vi "Main Loop.vi"(8 "error in (no error)":errorcluster, 10 "Chart Notifier":refnum<notifier>, 11 "Message Queues":T1) -> (0 "error out":errorcluster)   [LabVIEW 2018, in "Scale Module.lvlib" / "Scale Module Engine.lvlib"]
uses:
  Scale Module Engine.lvlib
  Scale Message Queues.ctl
  support/Message Queue/Message Cluster.ctl
  State Cluster.ctl
  State Enum.ctl
  Feed Module/Controls/Scale Module Settings Cluster.ctl
  Mettler Toledo/Controls/Settings Cluster.ctl
  Feed Module/Controls/Scale Module Display.ctl
  <vilib>/Platform/TimedLoop/XDataNode/timing_clust.ctl
  <vilib>/Platform/TimedLoop/XDataNode/nitl_modes.ctl
  <vilib>/Platform/TimedLoop/XDataNode/wakeup.ctl
  Tag VIs/Tag FGV Operation Enum.ctl
  support/Message Queue/Enqueue Message (Single).vi
  <vilib>/Platform/TimedLoop/XDataNode/XDataNode.xnode
  support/Message Queue/Message Queue.lvlib
  <vilib>/Platform/TimedLoop/XDataNode/XDNodeRunTimeDep.lvlib
  Scale Module.lvlib
  Mettler Toledo/Mettler Toledo.lvlib
  Shared Variables/Dynamic Shared Variables.lvlib
  support/Support Library.lvlib
panel:
  out "Period (s)":dbl format="%_4g"
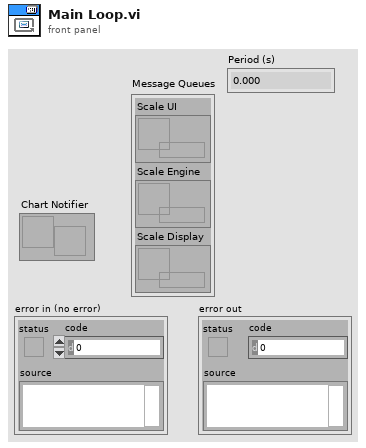
[diagram p1: front panel]
types:
  T1 = typedef "Scale Module.lvlib/Scale Message Queues.ctl" = cluster{"Scale UI":refnum<queue>, "Scale Engine":refnum<queue>, "Scale Display":refnum<queue>}
  T2 = typedef "Scale Module.lvlib/Scale Module Engine.lvlib/State Cluster.ctl" = cluster{"State":T3, "Start Time":timestamp, "Configuration":T4, "Current Time":timestamp, "First Iteration":bool, "Data":cluster{"Scale Read(g)":dbl}, "Process Name":string, "Log Started":bool}
  T3 = typedef "Scale Module.lvlib/Scale Module Engine.lvlib/State Enum.ctl" = enum16{"Measuring", "Idle"}
  T4 = typedef "Scale Module.lvlib/Scale Module Settings Cluster.ctl" = cluster{"Cycle Period":dbl, "Mettler":T5, "Scale Type":string}
  T5 = typedef "Mettler Toledo.lvlib/Settings Cluster.ctl" = cluster{"VISA resource name":refnum<visa-resource-name>, "Simulated?":bool}
  T6 = typedef "XDNodeRunTimeDep.lvlib/timing_clust.ctl" = cluster{"Expected End [f-1]":u64, "Actual End [f-1]":u64, "Finished Late? [f-1]":bool, "Expected End [i-1]":u64, "Actual End [i-1]":u64, "Finished Late? [i-1]":bool, "Expected Start [i]":u64, "Actual Start [i]":u64, "Expected Start [f]":u64, "Actual Start [f]":u64, "Source Name":string, "Structure Name":string, "Period":i64, "Deadline":i64, "Offset":i64, "Start":i64, "Priority":i32, "Timeout":i32, "Mode":T7, "Wakeup Reason":T8, "Error":errorcluster, "Source Type":string, "Secondary Source Type":string, "Global End Time":u64, "Global Start Time":u64, "Frame Duration":u64, "Iteration Duration":u64, "Assigned CPU":i32, "I/O Scan Engine Mode":u32}
  T7 = typedef "XDNodeRunTimeDep.lvlib/nitl_modes.ctl" = enum32{"No Change", "Process missed periods, maintain original phase", "Discard missed periods, maintain original phase", "Process missed periods, ignore original phase", "Discard missed periods, ignore original phase"}
  T8 = typedef "XDNodeRunTimeDep.lvlib/wakeup.ctl" = enum32{"Normal", "Aborted", "Asynchronous wakeup", "Timing source error", "Timed loop error", "Timeout"}
  T9 = cluster{"enable? (F)":bool, "name":string, "alarm on":bool, "priority":u32, "ack type":enum16{"Auto", "User", "None", "Each Occurrence"}, "area":string, "description":string, "log? (T)":bool}
  T10 = typedef "Tag FGV Operation Enum.ctl" = enum16{"Init", "Set Notification Queue", "Create Tag", "Commit", "Write Tag (Numeric)", "Write Tag (Boolean)", "Read All Tags", "Read One Tag", "Delete Tag Category", "Set Alarm Parameters (Numeric)", "Set Alarm Parameters (Boolean)", "Enable All Alarms", "Disable All Alarms", "Delete All Tags", "Read Alarms", "Ack Alarm", "Read Alarm Parameters (Numeric)", "Read Alarm Parameters (Boolean)"}
  T11 = enum32{"u32BitField", "bool", "double", "string", "int8", "uint8", "int16", "uint16", "int32", "uint32", "int64", "uint64", "single", "double waveform", "int16 waveform", "array of boolean", "array of int8", "array of uint8", "array of int16", "array of uint16", "array of int32", "array of uint32", "array of int64", "array of uint64", "array of single", "array of double", "array of double waveform", "array of int16 waveform", "array of string", "variant", "timestamp", "fixed point", "custom"}
  T12 = typedef "Scale Module.lvlib/Scale Module Display.ctl" = cluster{"Scale Value":dbl, "Cycle Period":dbl}
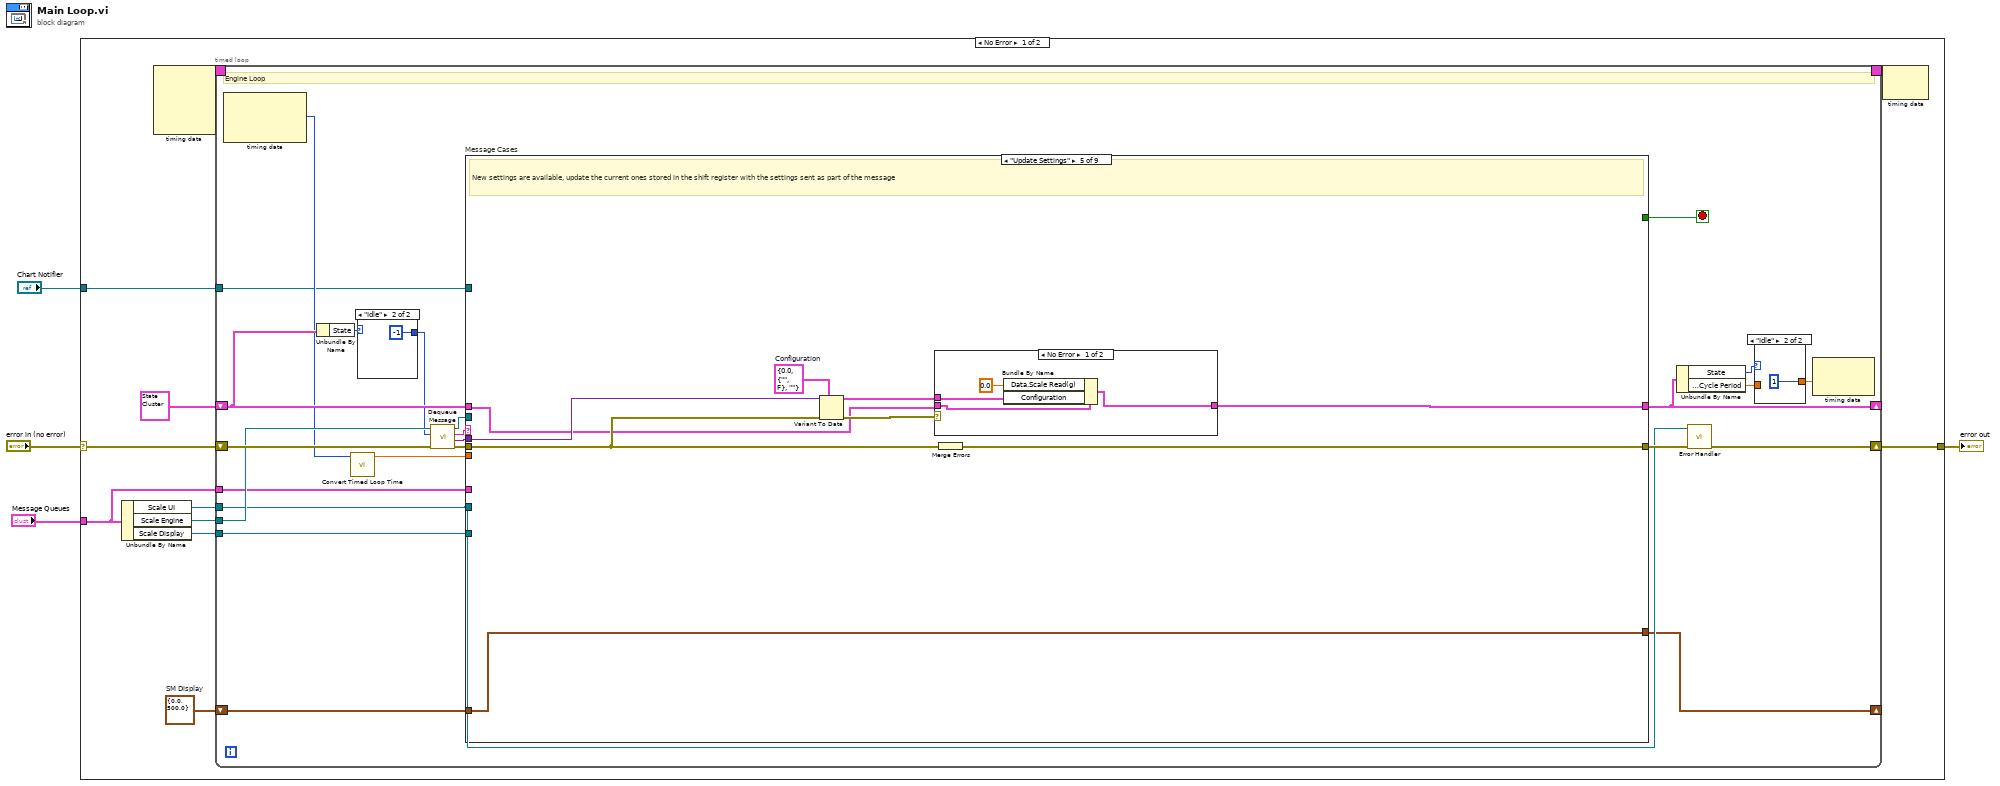
[diagram p0: block diagram]
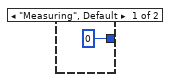
[diagram p3: hidden frame]
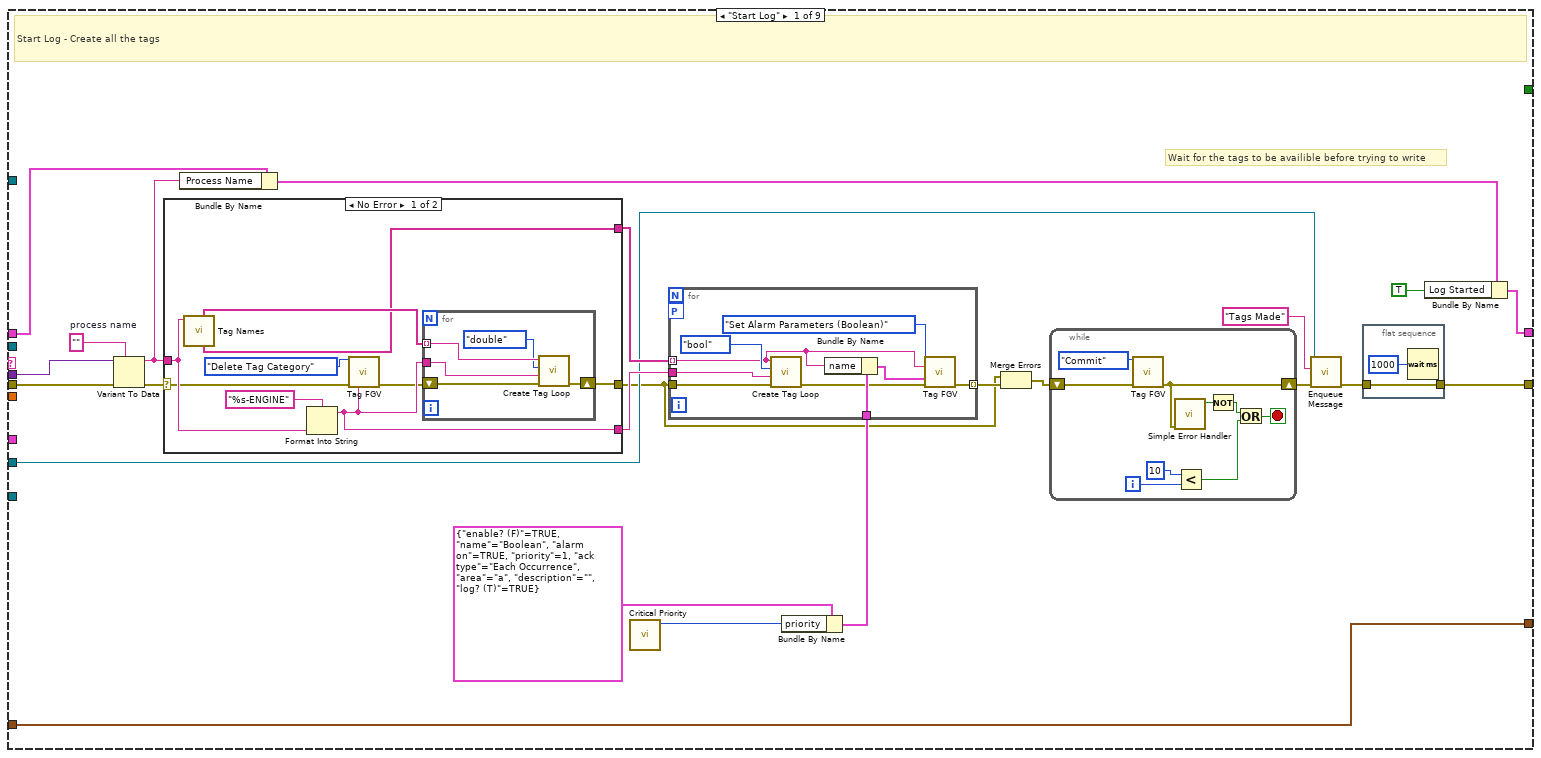
[diagram p4: hidden frame]
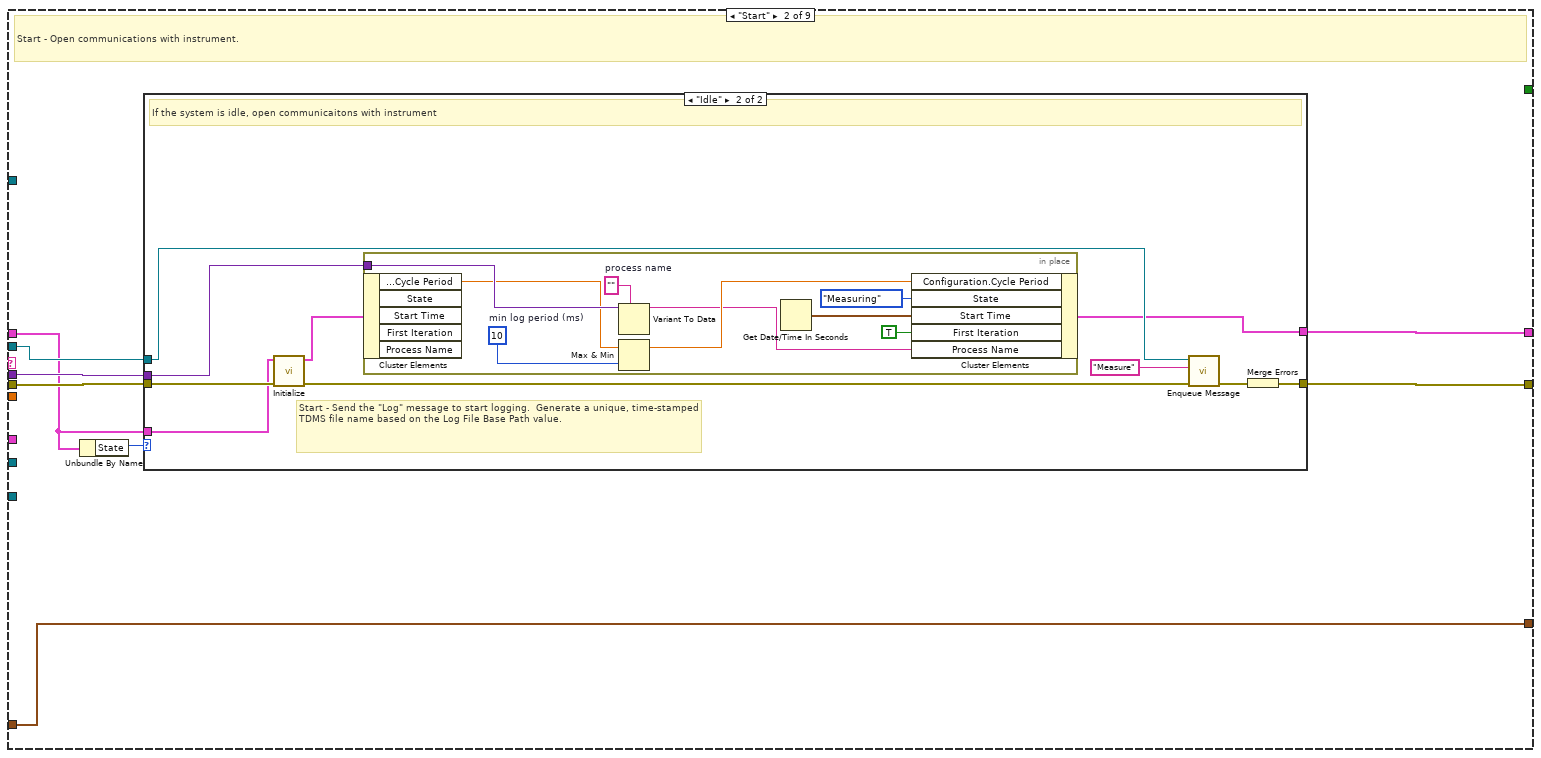
[diagram p6: hidden frame]
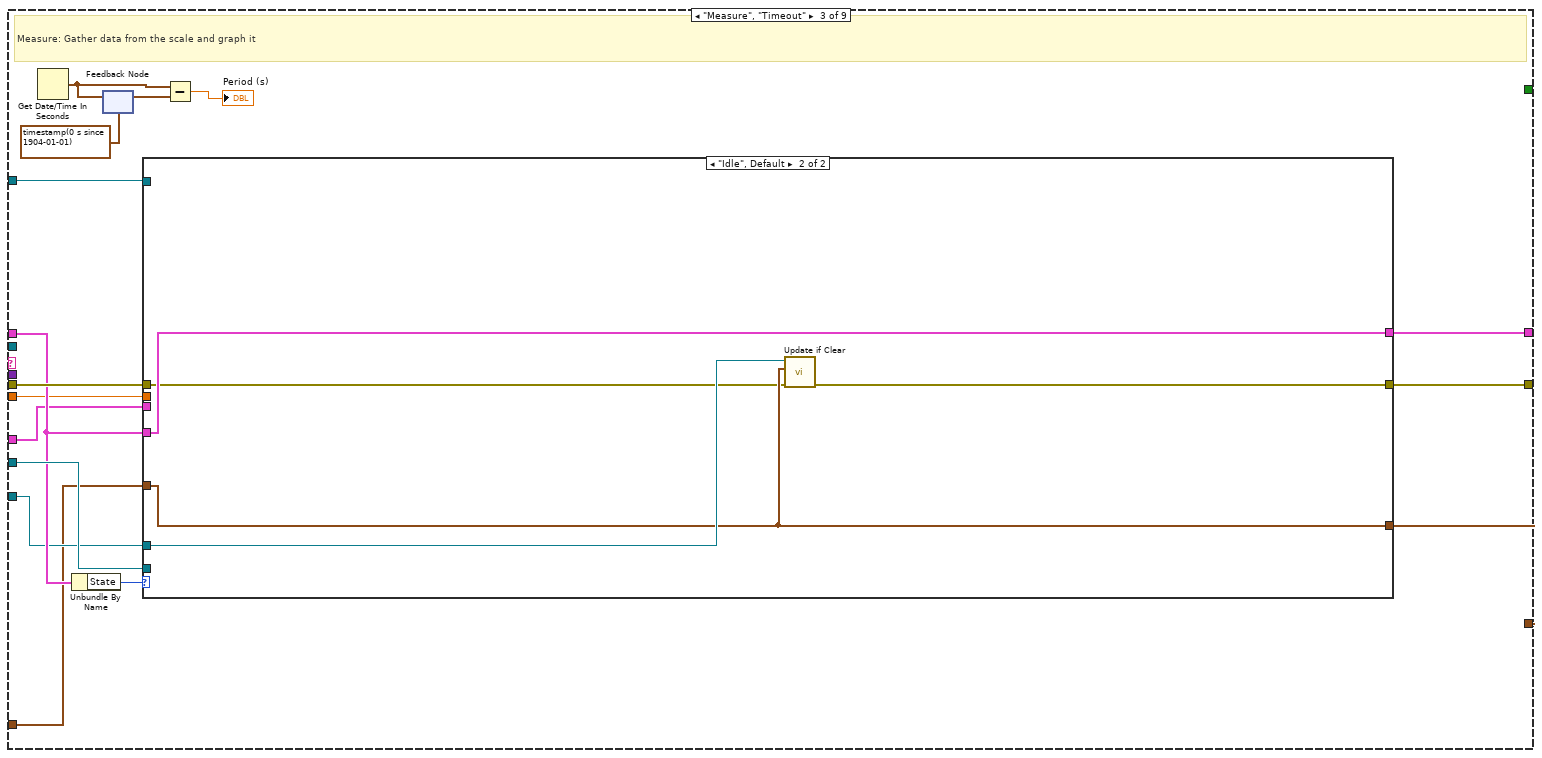
[diagram p8: hidden frame]
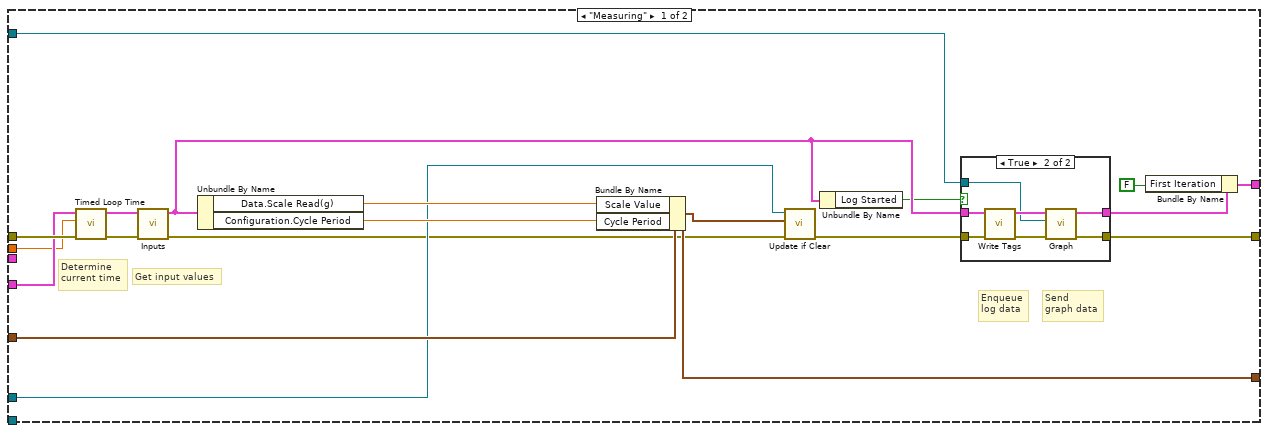
[diagram p9: hidden frame]
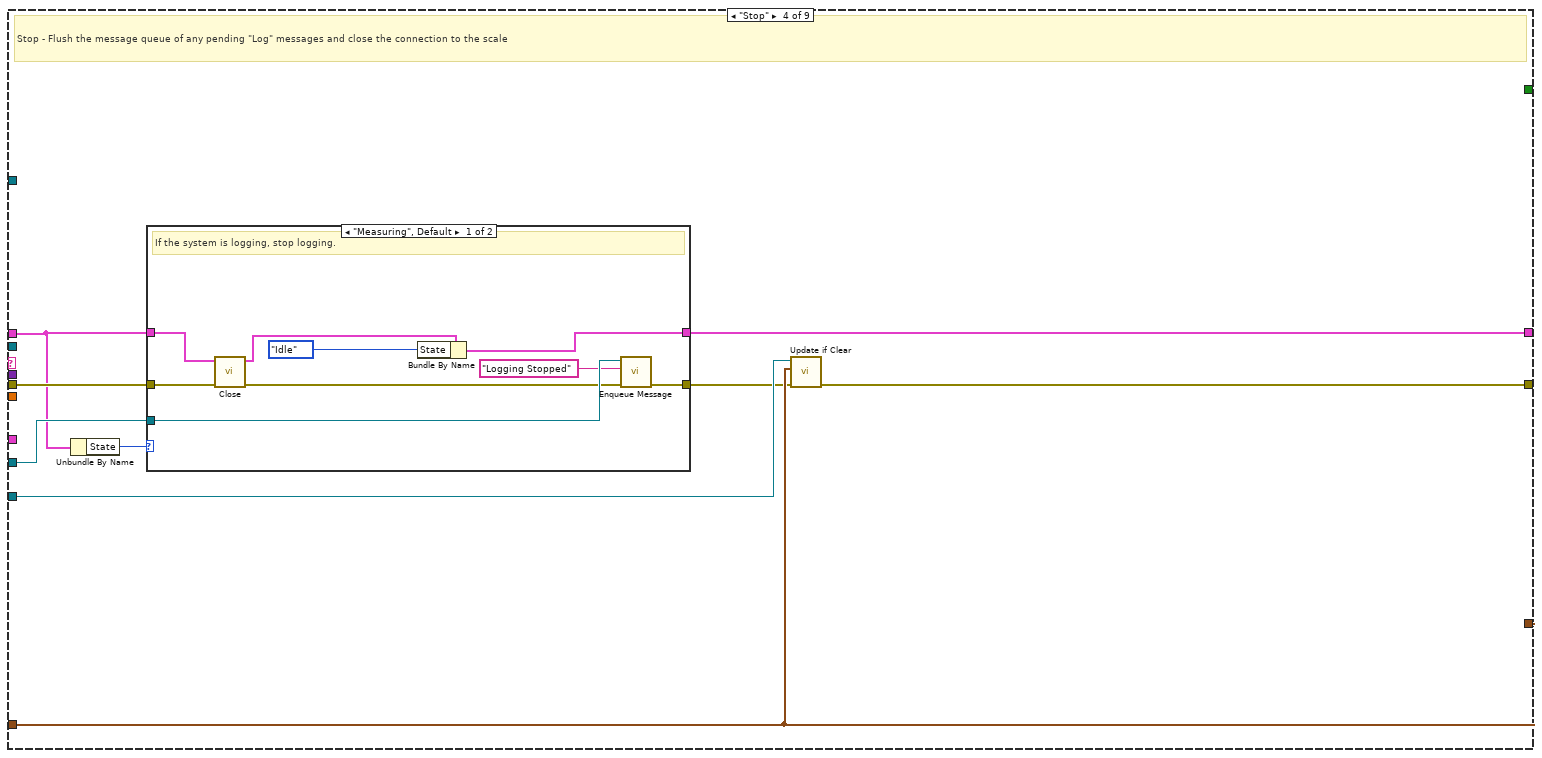
[diagram p11: hidden frame]
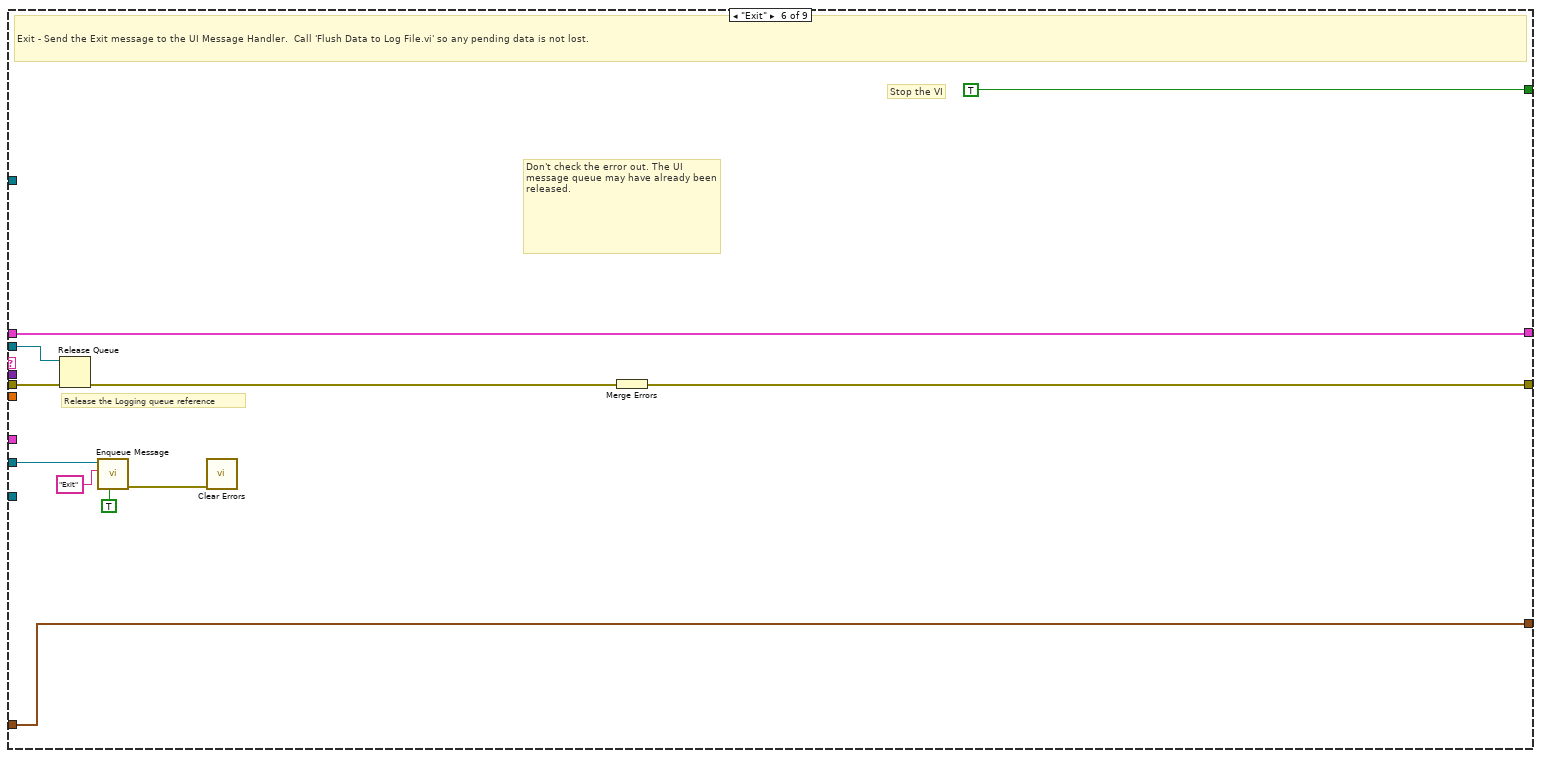
[diagram p14: hidden frame]
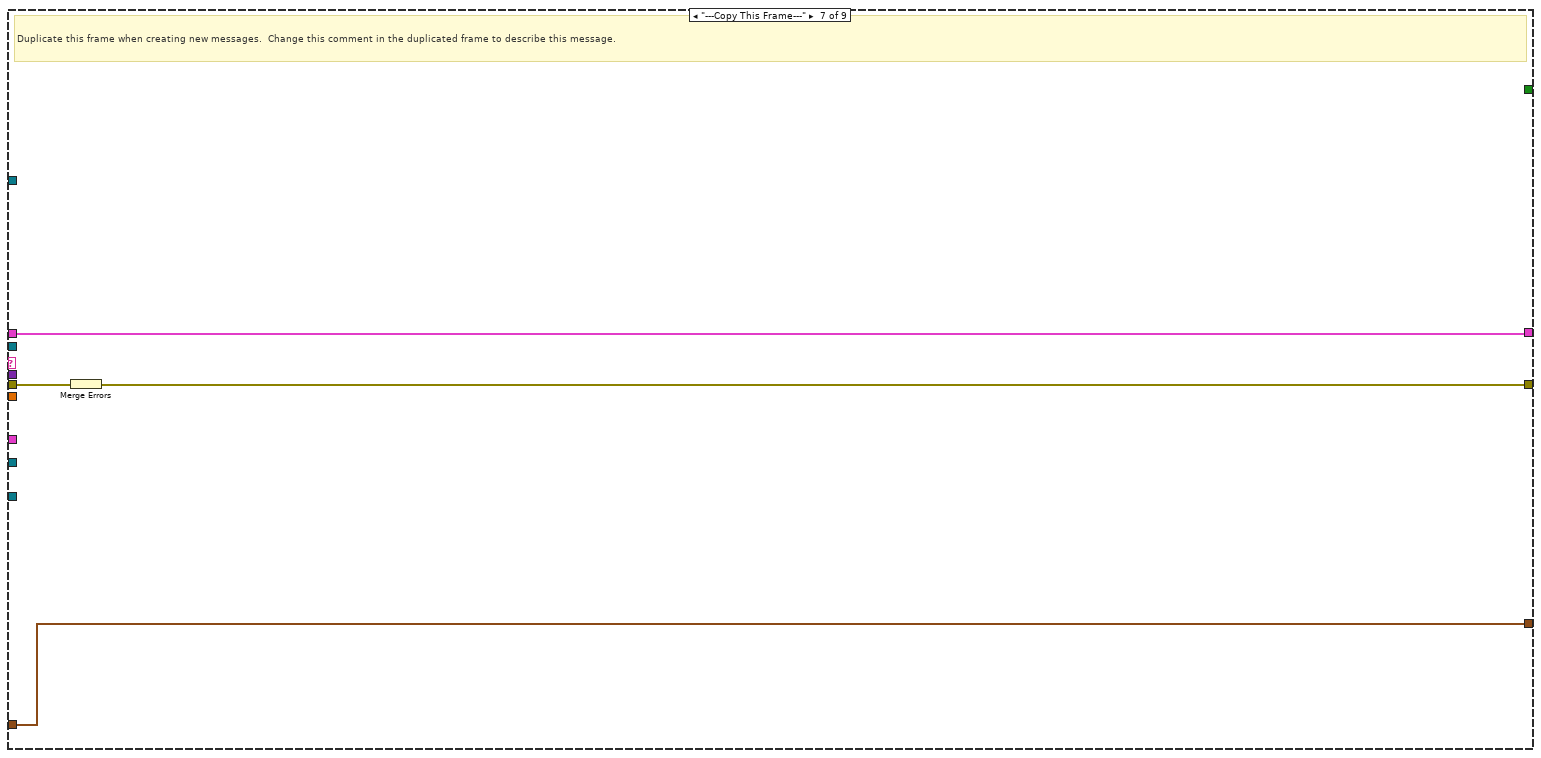
[diagram p15: hidden frame]
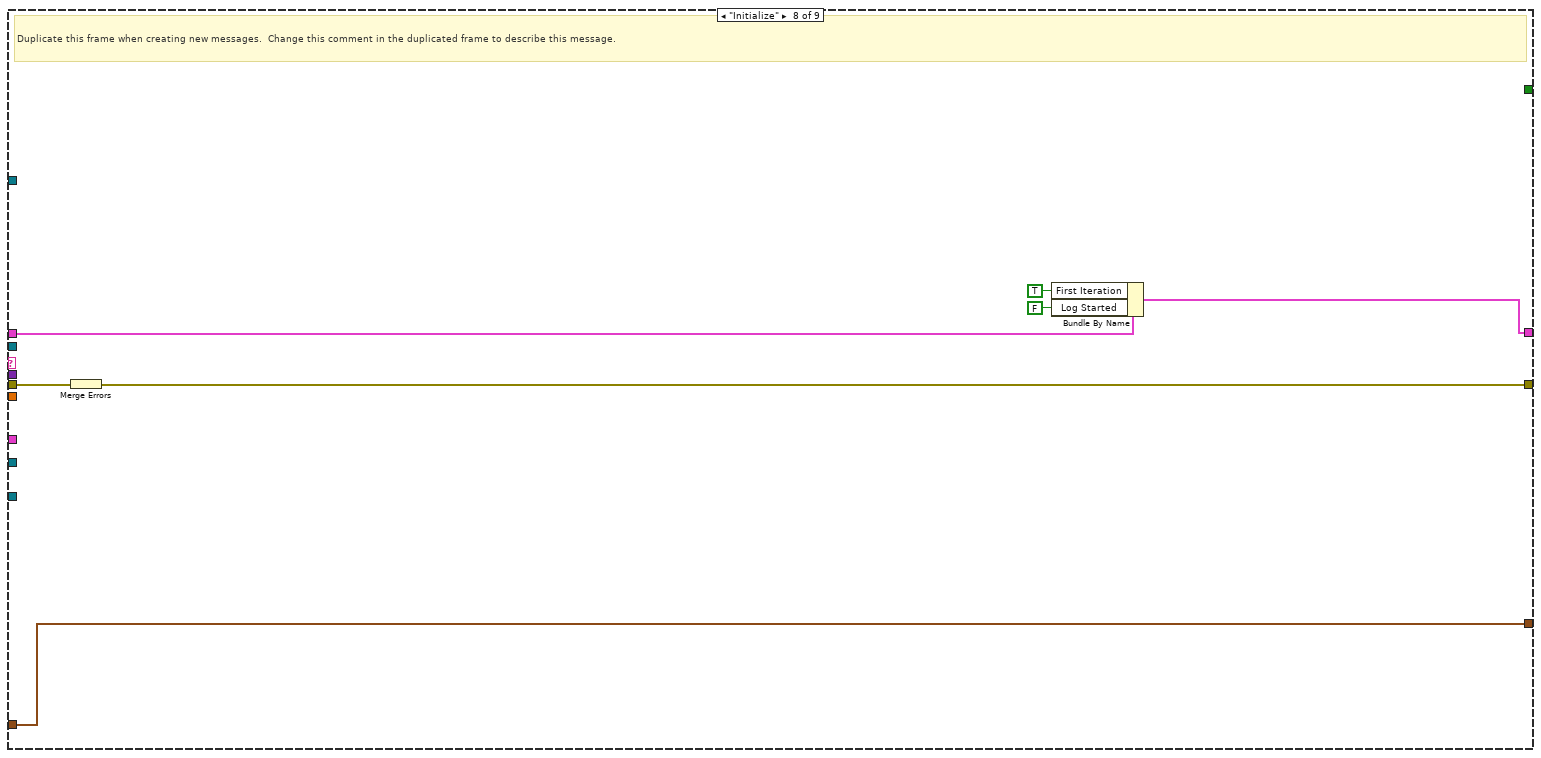
[diagram p16: hidden frame]
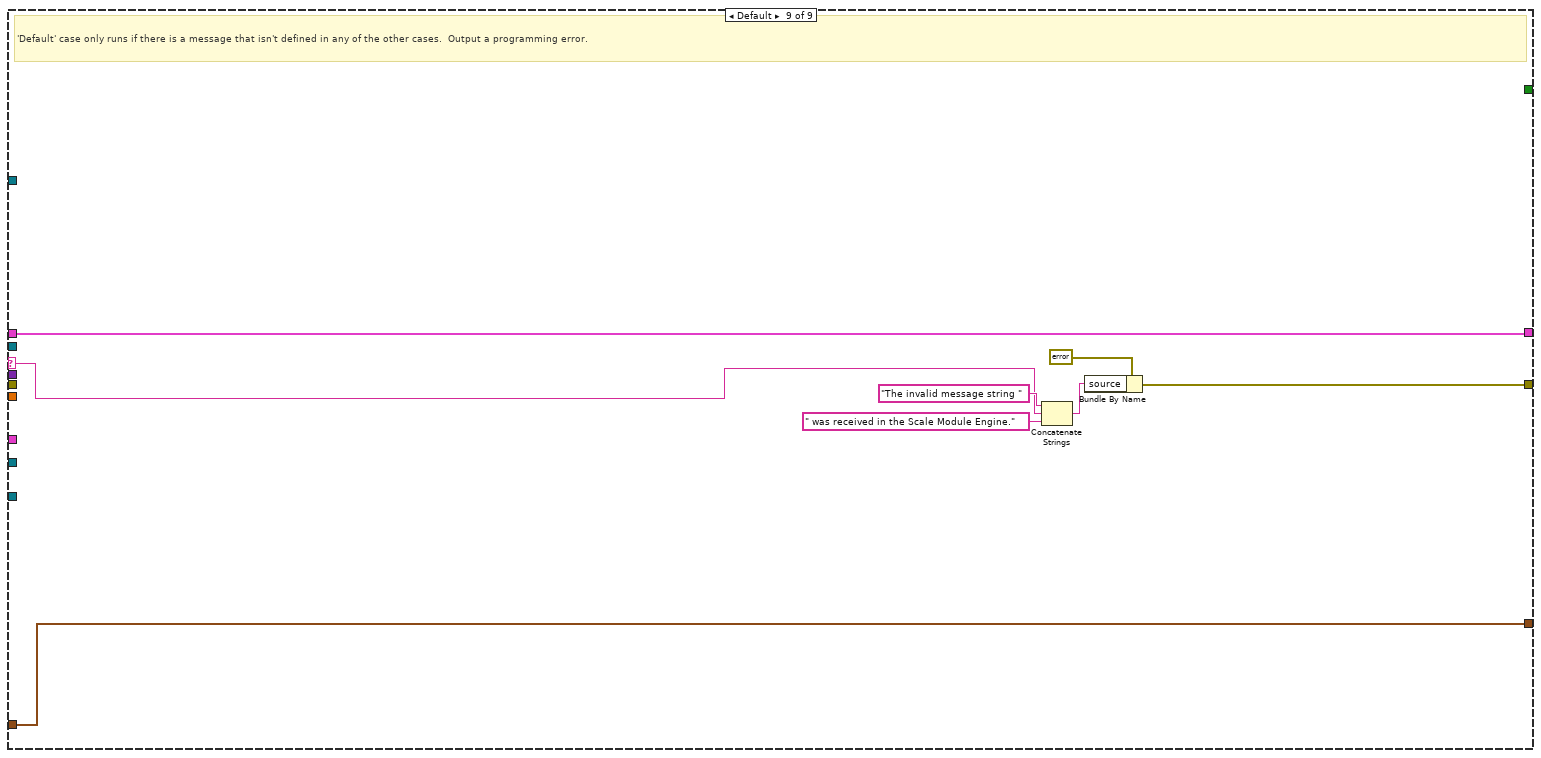
[diagram p17: hidden frame]
diagram:
  n1 = case shown="No Error" "error in (no error)" {
    selector: "error in (no error)" -> [w14 w251]
    tunnel: "Message Queues" -> [w9 _]
    tunnel: [w15 w251] -> w3
    tunnel: "Chart Notifier" -> [w7 _]
    frame No Error {
      w5 = T12 {"Scale Value"=0.0, "Cycle Period"=500.0}  # SM Display
      n2 = Unbundle By Name(w9) -> ("Scale UI"=w13:refnum<queue>, "Scale Engine"=w8:refnum<queue>, "Scale Display"=w6:refnum<queue>)
      n3 = node-c288() -> (w11:T6)  [unwired: 4 in]
      n4 = timed-loop {
        tunnel: w8 -> [w33]
        shift-right: [w17] -> _
        shift-left: T2 {"State"=enum."Idle", "Start Time"=timestamp(0 s since 1904-01-01), "Configuration"={"Cycle Period"=0.0, "Mettler"={"VISA resource name"="", "Simulated?"=FALSE}, "Scale Type"=""}, "Current Time"=timestamp(0 s since 1904-01-01), "First Iteration"=FALSE, "Data"={"Scale Read(g)"=0.0}, "Process Name"="", "Log Started"=FALSE} -> [w29]
        shift-right: [w31] -> w15
        shift-left: w14 -> [w38]
        tunnel: w13 -> [w30]
        timing: w11 -> [_]
        timing-out: [_] -> w10
        tunnel: w9 -> [w21]
        tunnel: w7 -> [w20]
        tunnel: w6 -> [w19]
        shift-right: [w18] -> _
        shift-left: w5 -> [w16]
        stop <- w39 stop-if-true
        # "Engine Loop"
        n5 = node-c288() -> (w23:i64)  [unwired: 1 in, 2 out]
        n6 = Unbundle By Name(w29) -> ("State"=w28:T3)
        n7 = call "Convert Timed Loop Time.vi"("Actual Start [i]"=w23) -> ("ET since start (s)"=w22:dbl)  [unwired: 10 in]
        n8 = case shown="\"Idle\"" w28 {
          tunnel: [0 ("timeout in ms (-1)") -1 ("timeout in ms (-1)")] -> w27
          frame "Measuring", Default {
          }
          frame "Idle" {
          }
        }
        n9 = call "Dequeue Message.vi"("error in (no error)"=w38, "timeout in ms (-1)"=w27, "Message Queue"=w33) -> ("error out"=w37:errorcluster, "Message Data"=w35:variant, "Message"=w36:string, "dup Message Queue"=w34:refnum<queue>)  [unwired: 5 in]
        n10 = case "Message Cases" shown="\"Update Settings\"" w36 {
          selector: w36 -> [_ _ _ _ _ _ _ _ w242]
          tunnel: w34 -> [_ w113 _ _ _ w223 _ _ _]
          tunnel: w37 -> [w66 w112 w148 w193 w211 w226 w233 w240 _]
          tunnel: [w50 w114 w149 w185 w213 w228 w232 w239 w241] -> w32
          tunnel: w29 -> [w65 w109 w147 w190 w209 w219 w230 w237 w247]
          tunnel: [_ _ _ _ _ TRUE _ _ _] -> w39
          tunnel: w35 -> [w67 w110 _ _ w212 _ _ _ _]
          tunnel: w30 -> [w54 _ w150 w192 _ w227 _ _ _]
          tunnel: w22 -> [_ _ w146 _ _ _ _ _ _]
          tunnel: w21 -> [_ _ w145 _ _ _ _ _ _]
          tunnel: w20 -> [_ _ w141 _ _ _ _ _ _]
          tunnel: w19 -> [_ _ w140 w188 _ _ _ _ _]
          tunnel: w16 -> [w71 w108 w139 w187 w206 w220 w231 w238 w248]
          tunnel: [w71 w108 w138 w187 w206 w220 w231 w238 w248] -> w18
          tunnel: [w57 w107 w137 w189 w205 w219 w230 w234 w247] -> w17
          frame "Start Log" {
            w70 = ""  # process name
            # "Wait for the tags to be availible before trying to write"
            # "Start Log - Create all the tags"
            n11 = Variant To Data(error in=w66, type=w70, Variant=w67) -> (data=w68:string, error out=w69:errorcluster)
            n12 = case shown="No Error" w69 {
              selector: w69 -> [w94 w106]
              tunnel: [w100 w106] -> w49
              tunnel: w68 -> [w98 _]
              tunnel: [w93 _] -> w61
              tunnel: [w96 _] -> w60
              frame No Error {
                n13 = call "Tag Names.vi"("Process Name"=w98) -> ("All Boolean Tags"=w96:string[], "All  Numeric Tags"=w97:string[])  [unwired: 8 in, 1 out]
                n14 = Format Into String(format string="%s-ENGINE", w98) -> (resulting string=w93:string)  [unwired: 2 in, 1 out]
                n15 = call "Tag FGV.vi"("Operation"=Tag_FGV_Operation_Enum."Delete Tag Category", "error in (no error)"=w94, "Tag Category"=w93) -> ("error out"=w92:errorcluster)  [unwired: 5 in, 7 out]
                n16 = for {
                  shift-right: [w105] -> w100
                  shift-left: w92 -> [w104]
                  tunnel: w93 -> [w101]
                  tunnel: w97 -> [w103] mode=indexing
                  n17 = call "Create Tag Loop.vi"("error in (no error)"=w104, "Tag Category"=w101, "data type"=T11."double", "Tag Name"=w103) -> ("error out"=w105:errorcluster)  [unwired: 7 in]
                }
              }
              frame Error {
              }
            }
            n18 = Bundle By Name(cluster=w65, "Process Name"=w68) -> (w58:T2)
            n19 = call "Critical Priority.vi"() -> ("critical priority"=w63:i32)  [unwired: 11 in]
            n20 = Bundle By Name(cluster=T9 {"enable? (F)"=TRUE, "name"="Boolean", "alarm on"=TRUE, "priority"=1, "ack type"=enum."Each Occurrence", "area"="a", "description"="", "log? (T)"=TRUE} ("Boolean alarm settings"), "priority"=w63) -> (w62:T9)
            n21 = for {
              tunnel: w62 -> [w91]
              tunnel: [w83] -> w59 mode=indexing
              tunnel: w60 -> [w85] mode=indexing
              tunnel: w61 -> [w88]
              tunnel: w49 -> [w90]
              workers-P: _ -> [_]
              n22 = call "Create Tag Loop.vi"("error in (no error)"=w90, "Tag Category"=w88, "data type"=T11."bool", "Tag Name"=w85) -> ("error out"=w84:errorcluster)  [unwired: 7 in]
              n23 = Bundle By Name(cluster=w91, "name"=w85) -> (w86:T9)
              n24 = call "Tag FGV.vi"("Operation"=Tag_FGV_Operation_Enum."Set Alarm Parameters (Boolean)", "Tag Name"=w85, "Data"=w86, "error in (no error)"=w84) -> ("error out"=w83:errorcluster)  [unwired: 4 in, 7 out]
            }
            n25 = Merge Errors(w49, w59) -> (w52:errorcluster)
            n26 = while {
              shift-right: [w74] -> w53
              shift-left: w52 -> [w75]
              i -> [w81]
              stop <- w77 stop-if-true
              n27 = call "Tag FGV.vi"("Operation"=Tag_FGV_Operation_Enum."Commit", "error in (no error)"=w75) -> ("error out"=w74:errorcluster)  [unwired: 6 in, 7 out]
              n28 = call <vilib>:"Simple Error Handler.vi"("error in (no error)"=w74) -> ("error?"=w82:bool)  [unwired: 4 in, 4 out]
              n29 = Less?(x=10, y=w81) -> (x < y?=w78:bool)
              n30 = Not(x=w82) -> (.not. x?=w79:bool)
              n31 = Or(x=w79, y=w78) -> (x .or. y?=w77:bool)
            }
            n32 = call-poly "Enqueue Message.vi"("error in (no error)"=w53, "Message"="Tags Made", "Message Queue"=w54) -> ("error out"=w51:errorcluster)  [unwired: 7 in, 1 out]
            n33 = flat-sequence {
              tunnel: [w72] -> w50
              tunnel: w51 -> [w72]
              frame #0 {
                n34 = Wait (ms)(milliseconds to wait=u32 1000) -> ()  [unwired: 1 out]
              }
            }
            n35 = Bundle By Name(cluster=w58, "Log Started"=TRUE) -> (w57:T2)
          }
          frame "Start" {
            # "Start - Open communications with instrument."
            n36 = Unbundle By Name(w109) -> ("State"=w111:T3)
            n37 = case shown="\"Idle\"" w111 {
              tunnel: [w115 w126] -> w114
              tunnel: w113 -> [_ w123]
              tunnel: w112 -> [w115 w121]
              tunnel: w109 -> [w116 w120]
              tunnel: [w116 w117] -> w107
              tunnel: w110 -> [_ w119]
              frame "Measuring", Default {
                # "The system is already running. Ignore the \"Start\" message."
              }
              frame "Idle" {
                # "Start - Send the \"Log\" message to start logging.  Generate a unique, time-stamped TDMS file name based on the Log File Base Path value."
                # "If the system is idle, open communicaitons with instrument"
                n38 = call "Initialize.vi"("error in (no error)"=w121, "State in"=w120) -> ("error out"=w122:errorcluster, "State out"=w118:T2)  [unwired: 8 in]
                n39 = in-place {
                  in-place-border: w119 -> [w133]
                  w134 = ""  # process name
                  w135 = 10  # min log period (ms)
                  n40 = in-place-cluster #1(w118) -> ("Configuration.Cycle Period"=w132:dbl)  [unwired: 4 out]
                  n41 = Variant To Data(type=w134, Variant=w133) -> (data=w127:string)  [unwired: 1 in, 1 out]
                  n42 = Max & Min(x=w132, y=w135) -> (max(x,y)=w131:dbl)  [unwired: 1 out]
                  n43 = Get Date/Time In Seconds() -> (seconds since 1Jan1904=w129:timestamp)
                  n44 = in-place-cluster #1("Configuration.Cycle Period"=w131, "State"=State_Enum."Measuring", "Start Time"=w129, "First Iteration"=TRUE, "Process Name"=w127) -> (w117:T2)
                }
                n45 = call-poly "Enqueue Message.vi"("error in (no error)"=w122, "Message"="Measure", "Message Queue"=w123) -> ("error out"=w124:errorcluster)  [unwired: 7 in, 1 out]
                n46 = Merge Errors(w124) -> (w126:errorcluster)
              }
            }
          }
          frame "Measure", "Timeout" {
            # "Measure: Gather data from the scale and graph it"
            n47 = Get Date/Time In Seconds() -> (seconds since 1Jan1904=w143:timestamp)
            n48 = Unbundle By Name(w147) -> ("State"=w151:T3)
            n49 = feedback-in #2(w143) -> ()
            n50 = feedback #2(timestamp(0 s since 1904-01-01) ("seconds since 1Jan1904")) -> (w144:timestamp)
            n51 = case shown="\"Idle\", Default" w151 {
              tunnel: w148 -> [w168 w181]
              tunnel: w147 -> [w166 w184]
              tunnel: w150 -> [_ _]
              tunnel: [w170 w180] -> w149
              tunnel: [w163 w184] -> w137
              tunnel: w146 -> [w165 _]
              tunnel: w145 -> [_ _]
              tunnel: w141 -> [w161 _]
              tunnel: w140 -> [w155 w183]
              tunnel: w139 -> [w160 w182]
              tunnel: [w154 w182] -> w138
              frame "Measuring" {
                # "Determine\ncurrent time"
                # "Send\ngraph data"
                # "Enqueue\nlog data"
                # "Get input values"
                n52 = call "Timed Loop Time.vi"("error in (no error)"=w168, "ET since start (s)"=w165, "State in"=w166) -> ("error out"=w169:errorcluster, "State out"=w167:T2)  [unwired: 7 in]
                n53 = call "Inputs.vi"("error in (no error)"=w169, "State in"=w167) -> ("error out"=w153:errorcluster, "State out"=w157:T2)  [unwired: 8 in]
                n54 = Unbundle By Name(w157) -> ("Data.Scale Read(g)"=w159:dbl, "Configuration.Cycle Period"=w158:dbl)
                n55 = Bundle By Name(cluster=w160, "Scale Value"=w159, "Cycle Period"=w158) -> (w154:T12)
                n56 = call "Update if Clear.vi"("error in (no error)"=w153, "Message Data"=w154, "Queue in"=w155) -> ("error out"=w152:errorcluster)  [unwired: 8 in]
                n57 = Unbundle By Name(w157) -> ("Log Started"=w156:bool)
                n58 = case shown="True" w156 {
                  tunnel: [w171 w177] -> w170
                  tunnel: [w172 w176] -> w164
                  tunnel: w161 -> [_ w175]
                  tunnel: w157 -> [w172 w174]
                  tunnel: w152 -> [w171 w173]
                  frame False {
                  }
                  frame True {
                    n59 = call "Write Tags.vi"("error in (no error)"=w173, "State in"=w174) -> ("error out"=w178:errorcluster, "State out"=w179:T2)  [unwired: 8 in]
                    n60 = call "Graph.vi"("error in (no error)"=w178, "notifier out"=w175, "State in"=w179) -> ("error out"=w177:errorcluster, "State out"=w176:T2)  [unwired: 7 in]
                  }
                }
                n61 = Bundle By Name(cluster=w164, "First Iteration"=FALSE) -> (w163:T2)
              }
              frame "Idle", Default {
                n62 = call "Update if Clear.vi"("error in (no error)"=w181, "Message Data"=w182, "Queue in"=w183) -> ("error out"=w180:errorcluster)  [unwired: 8 in]
              }
            }
            n63 = Subtract(x=w143, y=w144) -> (x-y=→"Period (s)":dbl)
          }
          frame "Stop" {
            # "Stop - Flush the message queue of any pending \"Log\" messages and close the connection to the scale"
            n64 = Unbundle By Name(w190) -> ("State"=w191:T3)
            n65 = case shown="\"Measuring\", Default" w191 {
              tunnel: [w198 w204] -> w186
              tunnel: w193 -> [w195 w204]
              tunnel: w192 -> [w202 _]
              tunnel: w190 -> [w196 w203]
              tunnel: [w200 w203] -> w189
              frame "Measuring", Default {
                # "If the system is logging, stop logging."
                n66 = call "Close.vi"("error in (no error)"=w195, "State in"=w196) -> ("error out"=w194:errorcluster, "State out"=w197:T2)  [unwired: 8 in]
                n67 = Bundle By Name(cluster=w197, "State"=State_Enum."Idle") -> (w200:T2)
                n68 = call-poly "Enqueue Message.vi"("error in (no error)"=w194, "Message"="Logging Stopped", "Message Queue"=w202) -> ("error out"=w198:errorcluster)  [unwired: 7 in, 1 out]
              }
              frame "Idle" {
                # "The system is already idle. Ignore the \"Stop\" message."
              }
            }
            n69 = call "Update if Clear.vi"("error in (no error)"=w186, "Message Data"=w187, "Queue in"=w188) -> ("error out"=w185:errorcluster)  [unwired: 8 in]
          }
          frame "Update Settings" {
            w207 = T4 {"Cycle Period"=0.0, "Mettler"={"VISA resource name"="", "Simulated?"=FALSE}, "Scale Type"=""}  # Configuration
            # "New settings are available, update the current ones stored in the shift register with the settings sent as part of the message"
            n70 = Variant To Data(error in=w211, type=w207, Variant=w212) -> (data=w208:T4, error out=w210:errorcluster)
            n71 = case shown="No Error" w210 {
              tunnel: w209 -> [w217 w218]
              tunnel: w208 -> [w216 _]
              tunnel: [w215 w218] -> w205
              frame No Error {
                n72 = Bundle By Name(cluster=w217, "Data.Scale Read(g)"=0.0, "Configuration"=w216) -> (w215:T2)
              }
              frame Error {
              }
            }
            n73 = Merge Errors(w211) -> (w213:errorcluster)
          }
          frame "Exit" {
            # "Release the Logging queue reference"
            # "Don't check the error out. The UI message queue may have already been released."
            # "Stop the VI"
            # "Exit - Send the Exit message to the UI Message Handler.  Call 'Flush Data to Log File.vi' so any pending data is not lost."
            n74 = Release Queue(queue=w223, error in (no error)=w226) -> (error out=w222:errorcluster)  [unwired: 1 in, 2 out]
            n75 = call-poly "Enqueue Message.vi"("Priority Message? (F)"=TRUE, "Message"="Exit", "Message Queue"=w227) -> ("error out"=w221:errorcluster)  [unwired: 7 in, 1 out]
            n76 = call <vilib>:"Clear Errors.vi"("error in (no error)"=w221) -> ()  [unwired: 5 in, 2 out]
            n77 = Merge Errors(w222) -> (w228:errorcluster)
          }
          frame "---Copy This Frame---" {
            # "Duplicate this frame when creating new messages.  Change this comment in the duplicated frame to describe this message."
            n78 = Merge Errors(w233) -> (w232:errorcluster)
          }
          frame "Initialize" {
            # "Duplicate this frame when creating new messages.  Change this comment in the duplicated frame to describe this message."
            n79 = Merge Errors(w240) -> (w239:errorcluster)
            n80 = Bundle By Name(cluster=w237, "First Iteration"=TRUE, "Log Started"=FALSE) -> (w234:T2)
          }
          frame Default {
            # "'Default' case only runs if there is a message that isn't defined in any of the other cases.  Output a programming error."
            n81 = Concatenate Strings("The invalid message string " ("string"), w242, " was received in the Scale Module Engine." ("string")) -> (w243:string)
            n82 = Bundle By Name(cluster=errorcluster {"status"=TRUE, "code"=1, "source"=""} ("error constant"), "source"=w243) -> (w241:errorcluster)
          }
        }
        n83 = Unbundle By Name(w17) -> ("State"=w26:T3, "Configuration.Cycle Period"=w24:dbl)
        n84 = call "Error Handler.vi"("error in (no error)"=w32, "Message Queue"=w30) -> ("dup error in"=w31:errorcluster)  [unwired: 8 in, 1 out]
        n85 = case shown="\"Idle\"" w26 {
          tunnel: [w40 1] -> w25
          tunnel: w24 -> [w40 _]
          frame "Measuring" {
          }
          frame "Idle" {
          }
        }
        n86 = node-c288(w25) -> ()  [unwired: 1 in, 1 out]
      }
      n87 = node-c288(w10) -> ()  [unwired: 1 out]
    }
    frame Error {
    }
  }
  "error out" <- w3
